vi "get auto box.vi"() -> (0 "Shoot During Autonomous?":bool, 1 "Use Hot Goal?":bool, 2 "2 Ball Autonomous?":bool, 3 "Disable Vison After Auto?":bool)   [LabVIEW 2014]
panel:
  # "Read Dashboard Auto Configuration"
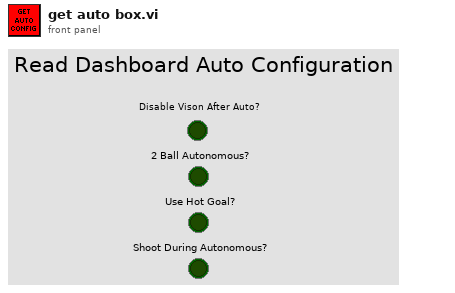
[diagram p1: front panel]
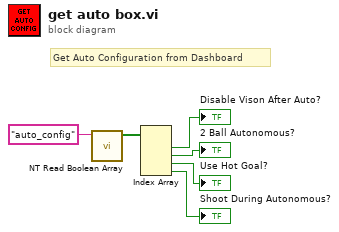
[diagram p0: block diagram]
diagram:
  # "Get Auto Configuration from Dashboard"
  n1 = call <vilib>:"NT Read Boolean Array.vi"("Name"="auto_config") -> ("Boolean Array"=w5:bool[])  [unwired: 9 in, 1 out]
  n2 = Index Array(array=w5) -> (element #1=→"Disable Vison After Auto?":bool, element #2=→"2 Ball Autonomous?":bool, element #3=→"Use Hot Goal?":bool, element #4=→"Shoot During Autonomous?":bool)  [unwired: 4 in]
